vi "Live window-Capture sliders distance.vi"(9 "Locked?":bool, 11 "Function":T1) -> ()   [LabVIEW 2013]
uses:
  Typedefs/Left-Right enum.ctl
  Globals/gl_Windows Ctrl refs.vi
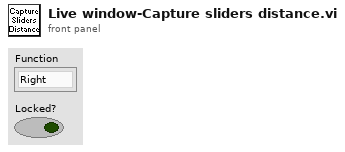
[diagram p1: front panel]
types:
  T1 = typedef "Left-Right enum.ctl" = enum16{"Right", "Left"}
  T2 = typedef "Live window-ctrl refs.ctl" = cluster{"This VI":refnum<vi>, "Pane":refnum<vi>, "Snapshot":refnum<vi>, "Left Image Palette":refnum<vi>, "Right Image Palette":refnum<vi>, "Left Channel":refnum<vi>, "Right Channel":refnum<vi>, "Left image intensity":refnum<vi>, "Right image intensity":refnum<vi>, "Left Image Display":T3, "Right Image Display":T3, "Refresh rate ind (Hz)":refnum<vi>, "Acq rate ind (Hz)":refnum<vi>, "Stop (ind)":refnum<vi>}
  T3 = typedef "Image display ref.ctl" = refnum<vi>
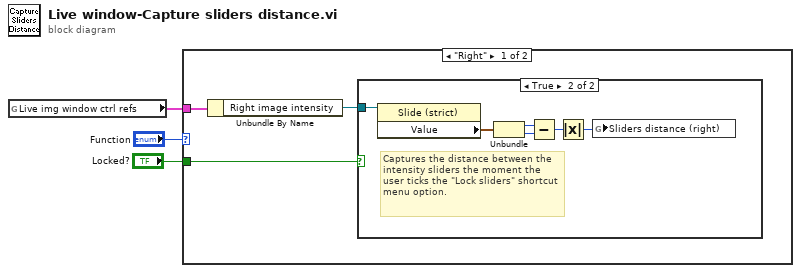
[diagram p0: block diagram]
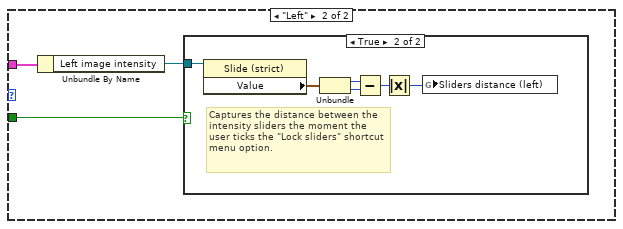
[diagram p3: hidden frame]
diagram:
  n1 = global read "gl_Windows Ctrl refs.vi" "Live img window ctrl refs"() -> (w1:T2)
  n2 = case shown="\"Right\"" "Function" {
    tunnel: w1 -> [w6 w15]
    tunnel: "Locked?" -> [w4 w13]
    frame "Right" {
      n3 = Unbundle By Name(w6) -> ("Right image intensity"=w5:refnum<vi>)
      n4 = case shown="True" w4 {
        tunnel: w5 -> [_ w8]
        frame False {
        }
        frame True {
          # "Captures the distance between the intensity sliders the moment the user ticks the \"Lock sliders\" shortcut menu option."
          n5 = property class="Slide (strict)"(reference=w8) -> ("Value"=w12:cluster{i16, i16})  [unwired: 1 in, 2 out]
          n6 = Unbundle(w12) -> (w11:i16, w7:i16)
          n7 = Subtract(x=w11, y=w7) -> (x-y=w10:i16)
          n8 = Absolute Value(x=w10) -> (abs(x)=w9:i16)
          n9 = global write "gl_Windows Ctrl refs.vi" "Sliders distance (right)"(w9) -> ()
        }
      }
    }
    frame "Left" {
      n10 = Unbundle By Name(w15) -> ("Left image intensity"=w14:refnum<vi>)
      n11 = case shown="True" w13 {
        tunnel: w14 -> [_ w17]
        frame False {
        }
        frame True {
          # "Captures the distance between the intensity sliders the moment the user ticks the \"Lock sliders\" shortcut menu option."
          n12 = property class="Slide (strict)"(reference=w17) -> ("Value"=w21:cluster{i16, i16})  [unwired: 1 in, 2 out]
          n13 = Unbundle(w21) -> (w20:i16, w16:i16)
          n14 = Subtract(x=w20, y=w16) -> (x-y=w19:i16)
          n15 = Absolute Value(x=w19) -> (abs(x)=w18:i16)
          n16 = global write "gl_Windows Ctrl refs.vi" "Sliders distance (left)"(w18) -> ()
        }
      }
    }
  }
